vi "Display One Button Popup.vi"(6 "Theme":refnum<class "Theme.lvclass">, 8 "error in":errorcluster, 10 "Message":string, 11 "Graphic":T1="info") -> (0 "error out":errorcluster)   [LabVIEW 2021, in "Pop-Up.lvlib" / "One Button.lvclass"]
doc: "The one button popup will display information to the user and wait for the operator to click the button.\n\n<b>Note:</b> The function <b>Close Pop-Up.vi</b> can be used to close this dialog early.\n\nInputs:\n-Graphic [typedef combobox] - Image (PNG) for Graphic for Popup\n-Message [String] - String Variable to populate Display\n-Theme [lvclass] - the theme for the style of the popup\n\n<b>Code Developed By:</b>\nDaniel Coons\nTechnology Service Corporation\n1983 S Liberty Drive\nBloomington, IN 47403\nPhone: 812 558-7100\ndaniel.coons@tsc.com\nwww.tsc.com/atcs"
uses:
  One Button.lvclass
  Theme/Theme.lvclass
  Graphics.ctl
  Pop-Up.lvlib
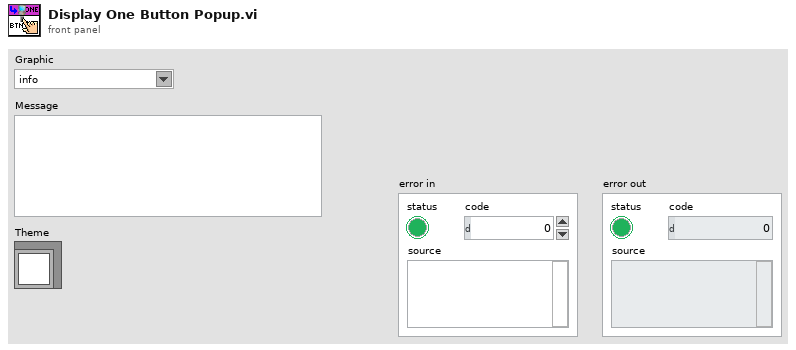
[diagram p1: front panel]
types:
  T1 = typedef "Pop-Up.lvlib/Graphics.ctl" = string
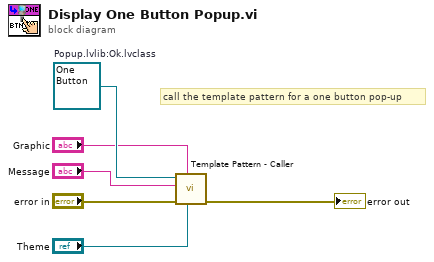
[diagram p0: block diagram]
diagram:
  w5 = refnum<class "One Button.lvclass"> refnum  # Popup.lvlib:Ok.lvclass
  # "call the template pattern for a one button pop-up"
  n1 = call-dynamic "Template Pattern - Caller.vi"("Theme"="Theme", "standard"="Graphic", "error in (no error)"="error in", "Message"="Message", "Pop-Up in"=w5) -> ("error out"=→"error out":errorcluster)  [unwired: 5 in, 1 out]
